vi "view.vi"(8 "error in (no error)":errorcluster, 9 "positionEvent":refnum<user-event>, 10 "AlCS.lvclass":refnum<class "AlCS.lvclass">, 11 "View in":refnum<class "View.lvclass">) -> (0 "error out":errorcluster, 3 "View out":refnum<class "View.lvclass">)   [LabVIEW 2016, in "View.lvclass"]
uses:
  View.lvclass
  AlCS/AlCS.lvclass
  AlCS/Subsystems.ctl
  AlCS/AlCS.lvclass/AlCS.ctl
  ts_labview_tcp/TCPCommunicator/TCPCommunicator.lvclass/TCPCommunicator.ctl
  ts_labview_tcp/TCPComEvents/TCPComEvents.lvclass/TCPComEvents.ctl
  ts_labview_tcp/TCPClient/TCPClient.lvclass
  home/andres/ts_alignmentsystemclient/ts_labview_tcp/TCPCommunicator/TCPCommunicator.lvclass
  ts_labview_tcp/TCPCommunicator/TCPCommunicator.lvclass
  ts_labview_tcp/TCPComEvents/TCPComEvents.lvclass
panel:
  out "Camera":T1(graph)
  out "M2":T1(graph)
  out "M1M3":T1(graph)
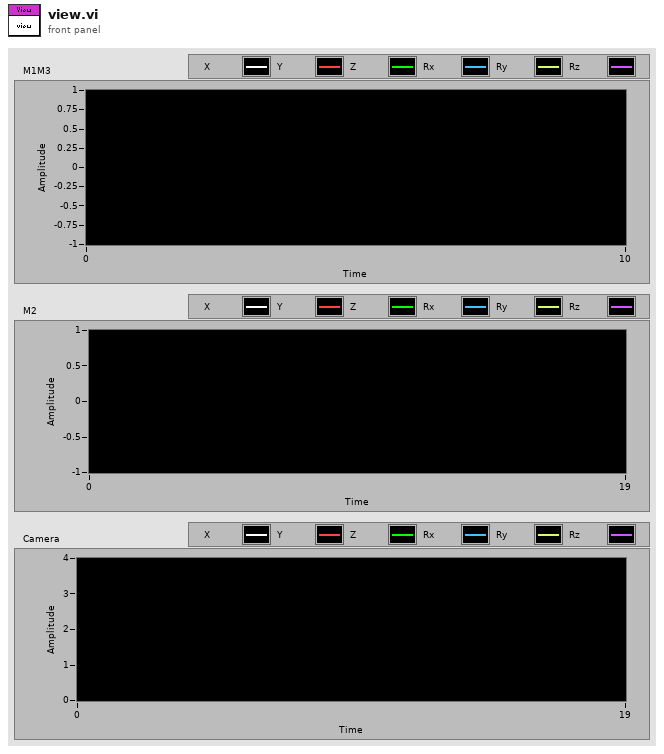
[diagram p1: front panel]
types:
  T1 = cluster{"x":dbl, "y":dbl, "z":dbl, "rx":dbl, "ry":dbl, "rz":dbl}
  T2 = typedef "Subsystems.ctl" = enum16{"M1M3", "Camera", "M2"}
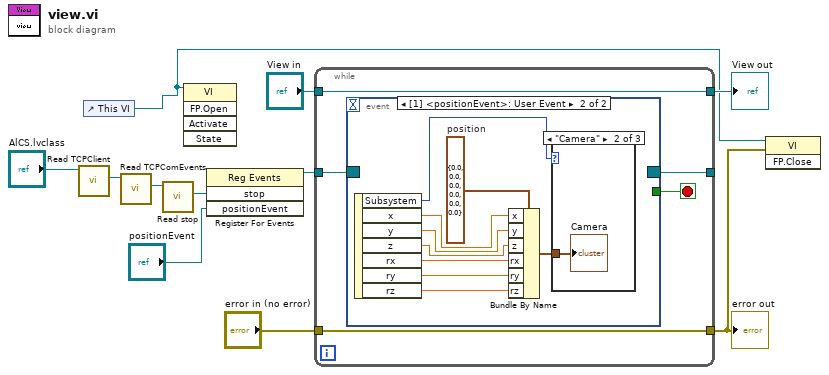
[diagram p0: block diagram]
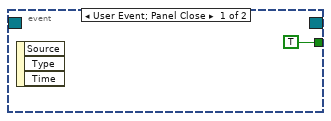
[diagram p2: hidden frame]
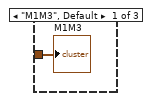
[diagram p3: hidden frame]
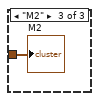
[diagram p4: hidden frame]
diagram:
  n1 = call "Read TCPClient.vi"("AlCS in"="AlCS.lvclass") -> ("TCPClient.lvclass"=w7:refnum<class "TCPClient.lvclass">)  [unwired: 8 in, 2 out]
  n2 = control-ref of="This VI"() -> (w2:refnum<vi>)
  n3 = call "Read TCPComEvents.vi"("TCPCommunicator in"=w7) -> ("TCPComEvents.lvclass"=w6:refnum<class "TCPComEvents.lvclass">)  [unwired: 8 in, 2 out]
  n4 = call "Read stop.vi"("TCPComEvents in"=w6) -> ("stop"=w5:refnum<user-event>)  [unwired: 8 in, 2 out]
  n5 = invoke class="VI" method="FP.Open"(reference=w2) -> ()  [unwired: 4 in, 5 out]
  n6 = register-events(w5, "positionEvent") -> (reference out=w4:refnum<event-registration>)  [unwired: 2 in, 1 out]
  n7 = while {
    tunnel: "View in" -> [w16]
    tunnel: [w16] -> w10
    tunnel: "error in (no error)" -> [w14]
    tunnel: [w14] -> w1
    tunnel: w4 -> [w13]
    tunnel: [w12] -> _
    stop <- w15 stop-if-true
    n8 = event shown="[1] <positionEvent>: User Event" {
      selector: w13 -> [_ _]
      dyn-events: [_ _] -> w12
      timeout: _ -> [_ _]
      tunnel: [TRUE ("stop") _] -> w15
      event User Event; Panel Close {
        n9 = event-data() -> ()  [unwired: 1 in, 3 out]
      }
      event User Event {
        w25 = T1 {"x"=0.0, "y"=0.0, "z"=0.0, "rx"=0.0, "ry"=0.0, "rz"=0.0}  # position
        n10 = event-data() -> ("Subsystem"=w26:T2, "x"=w24:dbl, "y"=w23:dbl, "z"=w22:dbl, "rx"=w21:dbl, "ry"=w20:dbl, "rz"=w19:dbl)  [unwired: 1 in]
        n11 = Bundle By Name(cluster=w25, "x"=w24, "y"=w23, "z"=w22, "rx"=w21, "ry"=w20, "rz"=w19) -> (w18:T1)
        n12 = case shown="\"Camera\"" w26 {
          tunnel: w18 -> [w27 w28 w29]
          frame "M1M3", Default {
            "M1M3" <- w27
          }
          frame "Camera" {
            "Camera" <- w28
          }
          frame "M2" {
            "M2" <- w29
          }
        }
      }
    }
  }
  "error out" <- w1
  "View out" <- w10
  n13 = invoke class="VI" method="FP.Close"(reference=w2, error in=w1) -> ()  [unwired: 1 in, 3 out]
